vi "Read Limit Switches.vi"(0 "LINX Resource":T1, 1 "Error In":errorcluster) -> (2 "LINX Resource 2":T1, 3 "Error Out":errorcluster, 4 "LS1":bool, 5 "LS2":bool, 6 "LS3":bool, 7 "LS4":bool)   [LabVIEW 2015]
uses:
  <vilib>/MakerHub/LINX/Private/Type Defs/LINX Ref.ctl
  <vilib>/MakerHub/LINX/Private/Type Defs/Platform.ctl
  <vilib>/MakerHub/LINX/Private/Type Defs/Interface.ctl
  <vilib>/MakerHub/LINX/Private/Device/Type Defs/LINX Device Config.ctl
  <vilib>/MakerHub/LINX/Private/Device/Type Defs/TCP Config.ctl
  <vilib>/MakerHub/LINX/Private/Device/Type Defs/Channels.ctl
  <vilib>/MakerHub/LINX/Public/Peripherals/Digital/Digital Read 1 Chan.vi
  <vilib>/MakerHub/LINX/LMH-LINX.lvlib
  <vilib>/MakerHub/LINX/Private/Device/Device.lvlib
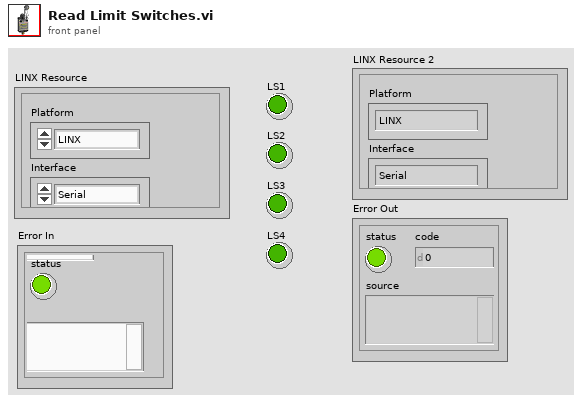
[diagram p1: front panel]
types:
  T1 = typedef "LMH-LINX.lvlib/LINX Ref.ctl" = cluster{"Platform":T2, "Interface":T3, "LINX Device Config":T4}
  T2 = typedef "LMH-LINX.lvlib/Platform.ctl" = enum16{"LINX", "myRIO"}
  T3 = typedef "LMH-LINX.lvlib/Interface.ctl" = enum16{"Serial", "TCP"}
  T4 = typedef "LMH-LINX.lvlib/Device.lvlib/LINX Device Config.ctl" = cluster{"Interface":T3, "COM Port":refnum<visa-resource-name>, "TCP Configuration":T5, "Device Family":u8, "Device ID":u8, "Device Name":string, "TCP Ref":refnum<k5>, "Channels":T6}
  T5 = typedef "LMH-LINX.lvlib/Device.lvlib/TCP Config.ctl" = cluster{"IP Address":string, "Port":u16}
  T6 = typedef "LMH-LINX.lvlib/Channels.ctl" = cluster{"DI":u8[], "DO":u8[], "AI":u8[], "AO":u8[], "PWM":u8[], "QE":u8[], "UART":u8[], "I2C 2":u8[], "SPI":u8[], "CAN":u8[], "Servo":u8[], "AI Ref (V)":dbl, "AO Ref (V)":dbl, "AO Resolution (Bits)":u8}
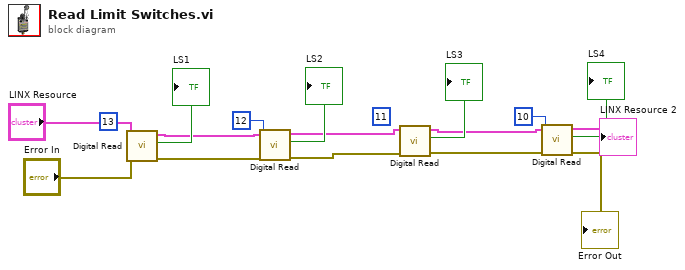
[diagram p0: block diagram]
diagram:
  (unwired) u8 11 ("DI Channel")
  n1 = call-poly <vilib>:"Digital Read.vi"("Error In"="Error In", "DI Channel"=u8 13, "LINX Resource"="LINX Resource") -> ("Error Out"=w7:errorcluster, "DI Value"=→"LS1":bool, "LINX Resource"=w8:T1)  [unwired: 6 in]
  n2 = call-poly <vilib>:"Digital Read.vi"("Error In"=w7, "DI Channel"=u8 12, "LINX Resource"=w8) -> ("Error Out"=w5:errorcluster, "DI Value"=→"LS2":bool, "LINX Resource"=w6:T1)  [unwired: 6 in]
  n3 = call-poly <vilib>:"Digital Read.vi"("Error In"=w5, "LINX Resource"=w6) -> ("Error Out"=w3:errorcluster, "DI Value"=→"LS3":bool, "LINX Resource"=w4:T1)  [unwired: 7 in]
  n4 = call-poly <vilib>:"Digital Read.vi"("Error In"=w3, "DI Channel"=u8 10, "LINX Resource"=w4) -> ("Error Out"=→"Error Out":errorcluster, "DI Value"=→"LS4":bool, "LINX Resource"=→"LINX Resource 2":T1)  [unwired: 6 in]
